vi "Actor.vi"(5 "Alias":string, 6 "Creator Attributes":refnum<class "Attributes.lvclass">, 9 "Queue of Self Attributes":refnum<queue>, 10 "Queue of Error":refnum<queue>, 11 "TEMPLATE Actor in":refnum<class "TEMPLATE Actor.lvclass">) -> (0 "Error out":errorcluster, 3 "TEMPLATE Actor out":refnum<class "TEMPLATE Actor.lvclass">)   [LabVIEW 2025, in "TEMPLATE Actor.lvlib" / "TEMPLATE Actor.lvclass"]
uses:
  TEMPLATE Actor.lvclass
  C:/Program Files/National Instruments/LabVIEW 2025/vi.lib/Nathan Davis/jettl/jettl/jettl/Actor/Actor/Actor.lvclass
  <vilib>/Nathan Davis/jettl/jettl/jettl/Attributes/Attributes/Attributes.lvclass
  Control Refs.ctl
  TEMPLATE Actor.lvclass/TEMPLATE Actor.ctl
  Update Pump State Msg/--direct.vi
  Update Pump State Msg/--created.vi
  Update Pump State Msg/--creator.vi
  Update Pump State Msg/--self.vi
  C:/git/jettl/message execution redesign/TEMPLATE Actor/TEMPLATE Actor/TEMPLATE Actor.lvclass
  C:/git/jettl/message execution redesign/Update Pump State Msg/Update Pump State/Update Pump State.lvclass
  <vilib>/Nathan Davis/jettl/jettl/jettl/Actor/Actor.lvlib
  Update Pump State Msg/Update Pump State Msg.lvlib
types:
  T1 = typedef "TEMPLATE Actor.lvlib/TEMPLATE Actor.lvclass/Control Refs.ctl" = cluster{"Placeholder":refnum<vi>}
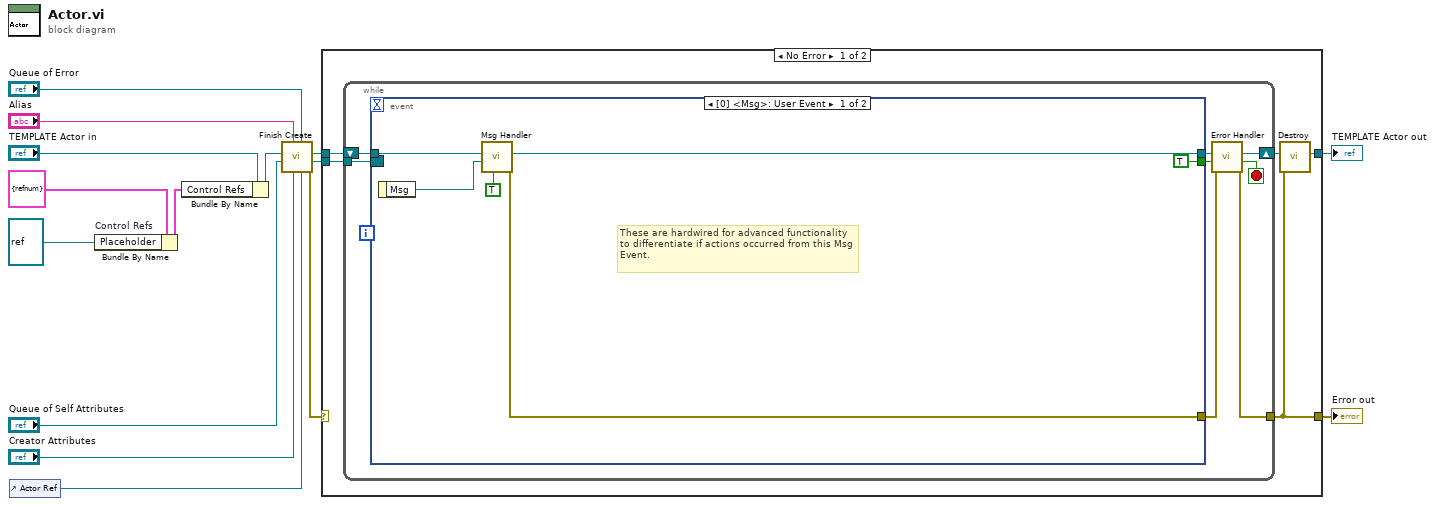
[diagram p0: block diagram]
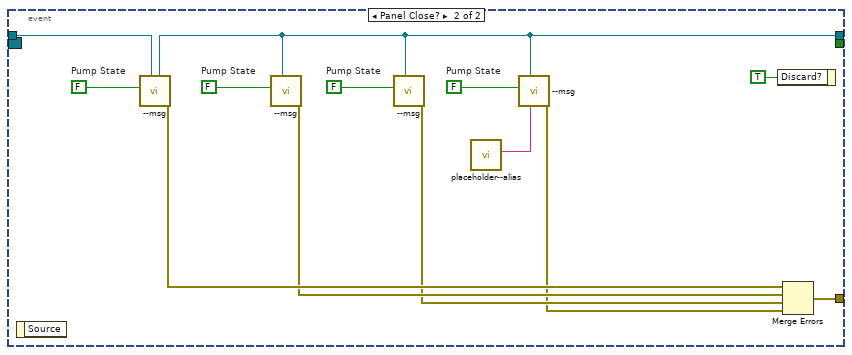
[diagram p2: hidden frame]
diagram:
  n1 = control-ref of="Actor Ref"() -> (w7:refnum<vi>)
  n2 = Bundle By Name "Control Refs"(cluster=T1 {"Placeholder"=refnum} ("Process Refs"), "Placeholder"=refnum<vi> refnum) -> (w13:T1)
  n3 = Bundle By Name(cluster="TEMPLATE Actor in", "Control Refs"=w13) -> (w9:refnum<class "TEMPLATE Actor.lvclass">)
  n4 = call <vilib>:"Finish Create.vi"("Actor Ref"=w7, "Queue of Error"="Queue of Error", "Creator Attributes"="Creator Attributes", "Alias"="Alias", "Queue of Self Attributes"="Queue of Self Attributes", "Actor in"=w9) -> ("Error out"=w3:errorcluster, "Event Ref"=w2:refnum<event-registration>, "Actor out"=w8:refnum<class "TEMPLATE Actor.lvclass">)  [unwired: 3 in]
  n5 = case shown="No Error" w3 {
    selector: w3 -> [_ w48]
    tunnel: [w18 w49] -> w15
    tunnel: w8 -> [w17 w49]
    tunnel: [w20 w48] -> w14
    tunnel: w2 -> [w16 _]
    frame No Error {
      n6 = while {
        shift-right: [w24] -> w19
        shift-left: w17 -> [w27]
        tunnel: w16 -> [w28]
        tunnel: [w22] -> w20
        stop <- w26 stop-if-true
        n7 = event shown="[0] <Msg>: User Event" {
          selector: w28 -> [_ _]
          dyn-events: _ -> [_ _]
          timeout: _ -> [_ _]
          tunnel: w27 -> [w33 w46]
          tunnel: [w31 w35] -> w25
          tunnel: [w34 w42] -> w23
          tunnel: [TRUE ("From Msg Event") _] -> w21
          event User Event {
            # "These are hardwired for advanced functionality to differentiate if actions occurred from this Msg Event."
            # "These are hardwired for advanced functionality to differentiate if actions occurred from this Msg Event."
            n8 = event-data() -> ("Msg"=w32:refnum<class "Msg.lvclass">)  [unwired: 1 in]
            n9 = call <vilib>:"Msg Handler.vi"("From Msg Event"=TRUE, "Msg"=w32, "Actor in"=w33) -> ("Error out"=w34:errorcluster, "Actor out"=w31:refnum<class "TEMPLATE Actor.lvclass">)  [unwired: 7 in]
          }
          event Panel Close? {
            w36 = FALSE  # Pump State
            w40 = FALSE  # Pump State
            w43 = FALSE  # Pump State
            w44 = FALSE  # Pump State
            n10 = event-data() -> ()  [unwired: 1 in, 1 out]
            n11 = call-poly "--msg.vi"("Actor in"=w46, "Pump State"=w44) -> ("Error out"=w45:errorcluster, "Actor out"=w35:refnum<class "TEMPLATE Actor.lvclass">)  [unwired: 8 in]
            n12 = call-poly "--msg.vi"("Actor in"=w35, "Pump State"=w43) -> ("Error out"=w41:errorcluster)  [unwired: 9 in]
            n13 = call-poly "--msg.vi"("Actor in"=w35, "Pump State"=w40) -> ("Error out"=w39:errorcluster)  [unwired: 9 in]
            n14 = call "placeholder--alias.vi"() -> ("Prefix"=w38:string)  [unwired: 11 in]
            n15 = call-poly "--msg.vi"("Alias"=w38, "Actor in"=w35, "Pump State"=w36) -> ("Error out"=w37:errorcluster)  [unwired: 8 in]
            n16 = event-data("Discard?"=TRUE) -> ()  [unwired: 1 in, 1 out]
            n17 = Merge Errors(w45, w41, w39, w37) -> (w42:errorcluster)
          }
        }
        n18 = call <vilib>:"Error Handler.vi"("Error in"=w23, "From Msg Event"=w21, "Actor in"=w25) -> ("Error out"=w22:errorcluster, "Destroy"=w26:bool, "Actor out"=w24:refnum<class "TEMPLATE Actor.lvclass">)  [unwired: 6 in]
      }
      n19 = call <vilib>:"Destroy.vi"("Error in"=w20, "Actor in"=w19) -> ("Actor out"=w18:refnum<class "TEMPLATE Actor.lvclass">)  [unwired: 9 in]
    }
    frame Error {
    }
  }
  "TEMPLATE Actor out" <- w15
  "Error out" <- w14
